vi "Remote Video stream (no write).vi"(1 "Quality":i32=750, 2 "Resolution":T1=1 items=["Low", "Med", "High", "Max."], 3 "Camera":T2="Travcam") -> (0 "Error out":errorcluster)   [LabVIEW 2015]
uses:
  Camera enum/Camera enum.ctl
  Camera enum/Camera resolution.ctl
  Globals/CamServer global.vi
panel:
  # "PN 27/08/15"
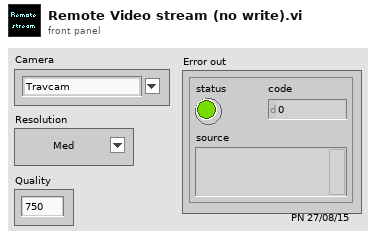
[diagram p1: front panel]
types:
  T1 = typedef "Camera resolution.ctl" = u8
  T2 = typedef "Camera enum.ctl" = string
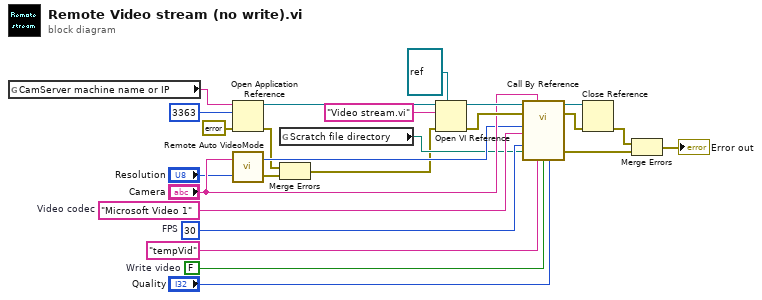
[diagram p0: block diagram]
diagram:
  w8 = "Microsoft Video 1"  # Video codec
  w9 = u32 30  # FPS
  w10 = FALSE  # Write video
  n1 = global read "CamServer global.vi" "CamServer machine name or IP"() -> (w7:string)
  n2 = Open Application Reference(8:errorcluster {"status"=FALSE, "code"=0, "source"=""} ("error in (no error)"), 10:u16 3363 ("port"), 11:w7) -> (0:w5:errorcluster, 3:w23:refnum<vi>)  [unwired: 1 in]
  n3 = call "Remote Auto VideoMode.vi"("Resolution"="Resolution", "Camera"="Camera") -> ("Error out"=w4:errorcluster, "VideoMode"=w13:u32)
  n4 = global read "CamServer global.vi" "Scratch file directory"() -> (w6:path)
  n5 = Merge Errors(w5, w4) -> (w3:errorcluster)
  n6 = Open VI Reference(type specifier VI Refnum (for type only)=refnum<vi> refnum, application reference (local)=w23, vi path="Video stream.vi" ("machine name"), error in (no error)=w3) -> (vi reference=w21:refnum<vi>, error out=w22:errorcluster)  [unwired: 2 in]
  n7 = call-by-ref "?"(reference=w21, error in=w22, "VideoMode"=w13, "Interface name"="Camera", "Video codec"=w8, "FPS"=w9, "Video directory path"=w6, "Video name"="tempVid" ("Image name"), "Write video"=w10, "Quality"="Quality") -> (reference out=w19:refnum<vi>, error out=w18:errorcluster, "Error Out"=w17:errorcluster)  [unwired: 7 in]
  n8 = Close Reference(reference=w19, error in (no error)=w18) -> (error out=w16:errorcluster)
  n9 = Merge Errors(w16, w17) -> (→"Error out":errorcluster)
